vi "Segment_d.vi"(11 "Input in Binary":bool[](array[boolean])) -> (3 "Segment d":bool)   [LabVIEW 2024]
panel:
  out "D":bool
  out "C":bool
  out "B":bool
  out "A":bool
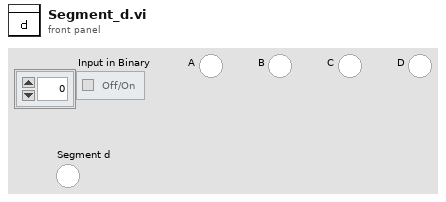
[diagram p1: front panel]
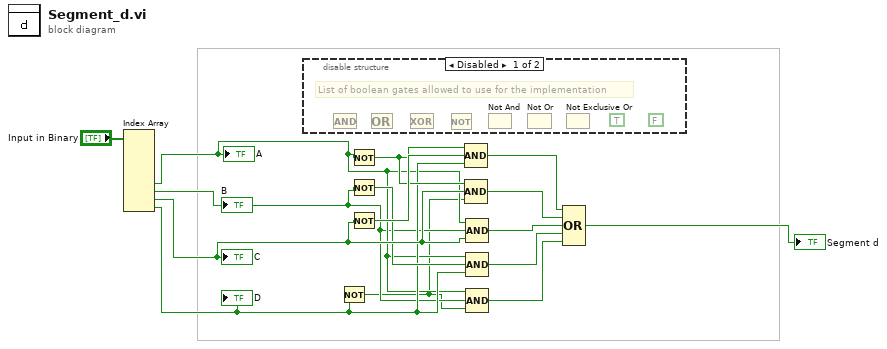
[diagram p0: block diagram]
diagram:
  n1 = Index Array(array="Input in Binary") -> (element #5=w9:bool, element #6=w8:bool, element #7=w12:bool, element #8=w10:bool)  [unwired: 8 in, 4 out]
  "A" <- w9
  "B" <- w8
  "C" <- w12
  "D" <- w10
  n2 = disable-structure shown="Disabled" {
    frame Disabled {
      (unwired) FALSE
      (unwired) TRUE
      # "List of boolean gates allowed to use for the implementation"
      n3 = And() -> ()  [unwired: 2 in, 1 out]
      n4 = Or() -> ()  [unwired: 2 in, 1 out]
      n5 = Exclusive Or() -> ()  [unwired: 2 in, 1 out]
      n6 = Not() -> ()  [unwired: 1 in, 1 out]
      n7 = Not And() -> ()  [unwired: 2 in, 1 out]
      n8 = Not Or() -> ()  [unwired: 2 in, 1 out]
      n9 = Not Exclusive Or() -> ()  [unwired: 2 in, 1 out]
    }
    frame Enabled {
    }
  }
  n10 = Not(x=w10) -> (.not. x?=w7:bool)
  n11 = Not(x=w9) -> (.not. x?=w13:bool)
  n12 = Not(x=w8) -> (.not. x?=w11:bool)
  n13 = Not(x=w12) -> (.not. x?=w14:bool)
  n14 = Compound Arithmetic op=AND(w13, w14, w10) -> (w1:bool)
  n15 = Compound Arithmetic op=AND(w13, w12, w7) -> (w2:bool)
  n16 = Compound Arithmetic op=AND(w9, w8, w12) -> (w3:bool)
  n17 = Compound Arithmetic op=AND(w9, w11, w10) -> (w4:bool)
  n18 = Compound Arithmetic op=AND(w9, w8, w7) -> (w5:bool)
  n19 = Compound Arithmetic op=OR(w1, w2, w3, w4, w5) -> (→"Segment d":bool)
